vi "Device.Uninit.vi"(8 "error in (no error)":errorcluster, 11 "XYStage.KIM101 in":refnum<class "XYStage.KIM101.lvclass">) -> (0 "error out":errorcluster, 3 "XYStage.KIM101 out":refnum<class "XYStage.KIM101.lvclass">)   [LabVIEW 2017, in "XYStage.KIM101.lvclass"]
uses:
  XYStage.KIM101.lvclass
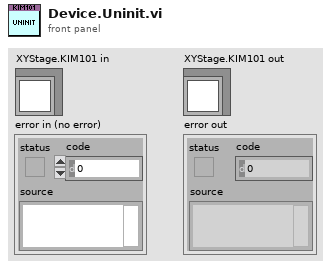
[diagram p1: front panel]
types:
  T1 = typedef "XYStage.KIM101.lvclass/Resource--Cluster.ctl" = cluster{"KCubeInertialMotorControl":refnum<k24>, "Device":refnum<k24>, "X Axis Channel":i32, "Y Axis Channel":i32}
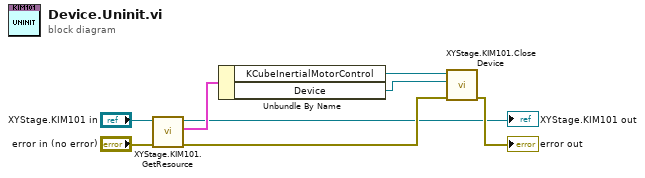
[diagram p0: block diagram]
diagram:
  n1 = call "XYStage.KIM101.GetResource.vi"("error in (no error)"="error in (no error)", "XYStage.KIM101 in"="XYStage.KIM101 in") -> ("error out"=w3:errorcluster, "Resource"=w6:T1, "XYStage.KIM101 out"=→"XYStage.KIM101 out":refnum<class "XYStage.KIM101.lvclass">)  [unwired: 7 in]
  n2 = Unbundle By Name(w6) -> ("KCubeInertialMotorControl"=w5:refnum<k24>, "Device"=w4:refnum<k24>)
  n3 = call "XYStage.KIM101.Close Device.vi"("error in (no error)"=w3, "Device"=w4, "KCubeInertialMotorControl in"=w5) -> ("error out"=→"error out":errorcluster)  [unwired: 8 in]
